vi "Create File.vi"(6 "Error in":errorcluster, 9 "File Name":path) -> (0 "Error out":errorcluster, 3 "file_id":i32)   [LabVIEW 2011, in "HDF5Tools.lvlib"]
uses:
  HDF5Tools.lvlib
  Release/HDF5Tools.dll
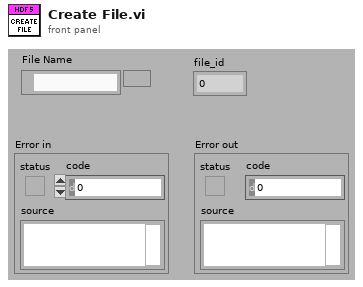
[diagram p1: front panel]
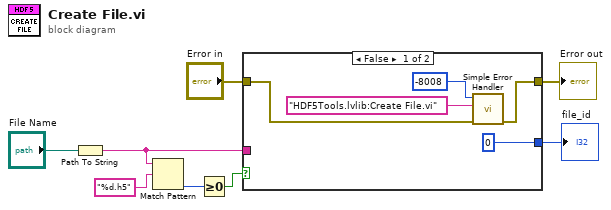
[diagram p0: block diagram]
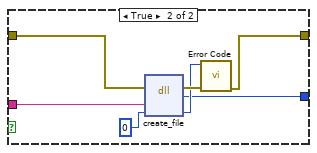
[diagram p2: hidden frame]
diagram:
  n1 = Path To String(path="File Name") -> (string=w6:string)
  n2 = Match Pattern(string=w6, regular expression="%d.h5" ("name")) -> (offset past match=w5:i32)  [unwired: 1 in, 3 out]
  n3 = Greater Or Equal To 0?(x=w5) -> (x >= 0?=w4:bool)
  n4 = case shown="False" w4 {
    tunnel: w6 -> [_ w17]
    tunnel: [0 ("file_id") w16] -> w3
    tunnel: "Error in" -> [w9 w15]
    tunnel: [w12 w14] -> w1
    frame False {
      n5 = call <vilib>:"Simple Error Handler.vi"("error code (no error:0)"=-8008, "error source (\" \")"="HDF5Tools.lvlib:Create File.vi" ("error source (\" \")"), "error in (no error)"=w9) -> ("error out"=w12:errorcluster)  [unwired: 2 in, 4 out]
    }
    frame True {
      n6 = dll-call lib="F:/HDF5Tools/Release/HDF5Tools.dll" fn="create_file"(error in=w15, "name"=w17, "error"=0) -> (error out=w19:errorcluster, "file_id"=w16:i32, "error"=w18:i32)  [unwired: 3 in, 1 out]
      n7 = call "Error Code.vi"("Error in"=w19, "Error code"=w18) -> ("Error out"=w14:errorcluster)  [unwired: 9 in]
    }
  }
  "file_id" <- w3
  "Error out" <- w1
